vi "Open Command Panel.vi"(9 "Cached Commands":T1, 10 "Commands":cluster{"Time (s)":dbl, T2, bool}[](array[cluster]), 11 "Tag":string) -> (3 "Found":bool)   [LabVIEW 2025]
uses:
  Types/Single Cmd Info.ctl
  <vilib>/picture/picture.llb/imagedata.ctl
  Types/Command Editor Info.ctl
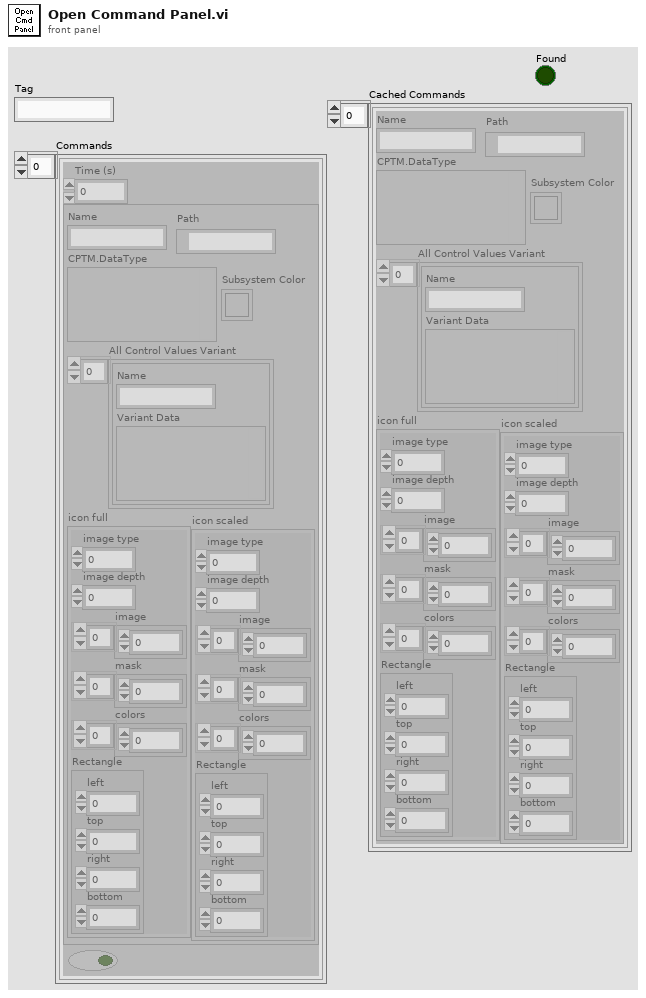
[diagram p1: front panel]
types:
  T1 = typedef "Command Editor Info.ctl" = T2[]
  T2 = typedef "Single Cmd Info.ctl" = cluster{"Name":string, "CPTM.DataType":variant, "All Control Values Variant":cluster{"Name":string, "Variant Data":variant}[], "icon full":T3, "icon scaled":T3, "Path":path, "Subsystem Color":u32}
  T3 = typedef "imagedata.ctl" = cluster{"image type":i32, "image depth":i32, "image":u8[], "mask":u8[], "colors":u32[], "Rectangle":cluster{"left":i16, "top":i16, "right":i16, "bottom":i16}}
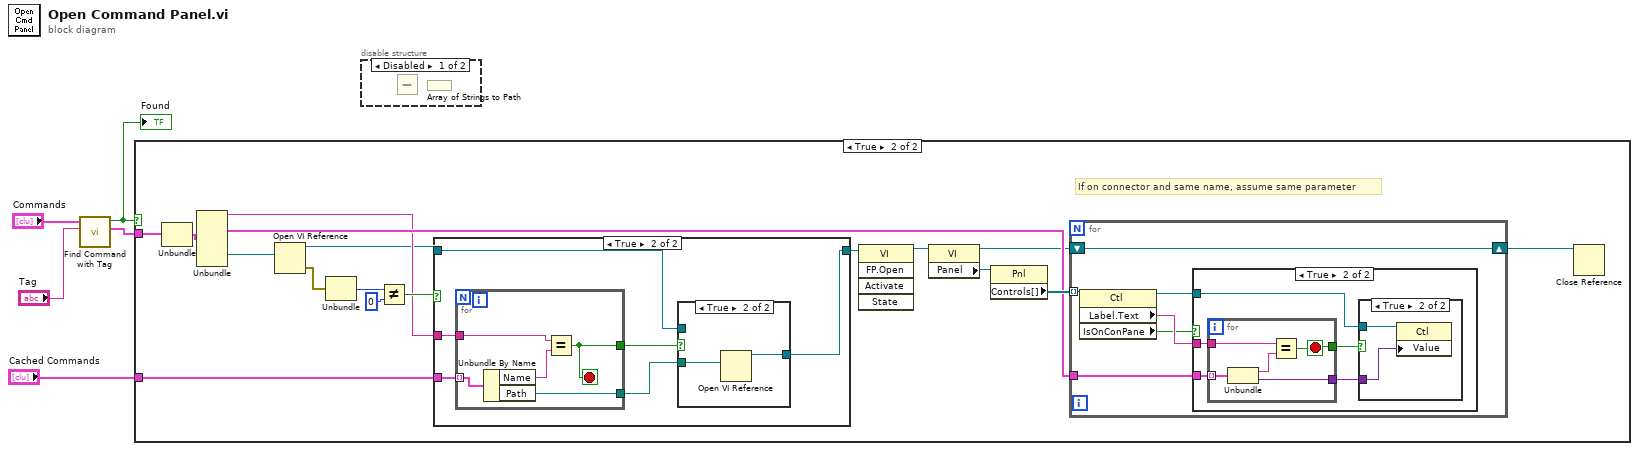
[diagram p0: block diagram]
diagram:
  n1 = call "Find Command with Tag.vi"("Command Tag"="Tag", "Commands"="Commands") -> ("Found Command"=w4:cluster{"Time (s)":dbl, T2, bool}, "Found"=w3:bool)  [unwired: 7 in, 1 out]
  "Found" <- w3
  n2 = case shown="True" w3 {
    tunnel: w4 -> [_ w22]
    tunnel: "Cached Commands" -> [_ w9]
    frame False {
    }
    frame True {
      # "If on connector and same name, assume same parameter"
      n3 = Unbundle(w22) -> (w21:T2)  [unwired: 2 out]
      n4 = Unbundle(w21) -> ("Name"=w8:string, "All Control Values Variant"=w17:cluster{"Name":string, "Variant Data":variant}[], "Path"=w11:path)  [unwired: 4 out]
      n5 = Open VI Reference(vi path=w11) -> (vi reference=w7:refnum<vi>, error out=w14:errorcluster)  [unwired: 5 in]
      n6 = Unbundle(w14) -> ("code"=w13:i32)  [unwired: 2 out]
      n7 = Not Equal?(x=w13, y=0) -> (x != y?=w10:bool)
      n8 = case shown="True" w10 {
        tunnel: w9 -> [_ w29]
        tunnel: w8 -> [_ w28]
        tunnel: w7 -> [w23 w24]
        tunnel: [w23 w25] -> w6
        frame False {
        }
        frame True {
          n9 = for {
            tunnel: w29 -> [w37] mode=indexing
            tunnel: w28 -> [w35]
            tunnel: [w34] -> w27
            tunnel: [w33] -> w26
            stop <- w34 stop-if-true
            n10 = Unbundle By Name(w37) -> ("Name"=w36:string, "Path"=w33:path)
            n11 = Equal?(x=w35, y=w36) -> (x = y?=w34:bool)
          }
          n12 = case shown="True" w27 {
            tunnel: w26 -> [_ w32]
            tunnel: [w30 w31] -> w25
            tunnel: w24 -> [w30 _]
            frame False {
            }
            frame True {
              n13 = Open VI Reference(vi path=w32) -> (vi reference=w31:refnum<vi>)  [unwired: 5 in, 1 out]
            }
          }
        }
      }
      n14 = invoke class="VI" method="FP.Open"(reference=w6) -> (reference out=w19:refnum<vi>)  [unwired: 4 in, 4 out]
      n15 = property class="VI"(reference=w19) -> (reference out=w16:refnum<vi>, "Panel"=w20:refnum<vi>)  [unwired: 1 in, 1 out]
      n16 = property class="Pnl"(reference=w20) -> ("Controls[]"=w18:refnum<vi>[])  [unwired: 1 in, 2 out]
      n17 = for {
        tunnel: w18 -> [w42] mode=indexing
        tunnel: w17 -> [w43]
        shift-right: [w38] -> w15
        shift-left: w16 -> [w38]
        n18 = property class="Ctl"(reference=w42) -> (reference out=w39:refnum<vi>, "Label.Text"=w41:string, "IsOnConPane"=w40:bool)  [unwired: 1 in, 1 out]
        n19 = case shown="True" w40 {
          tunnel: w43 -> [_ w48]
          tunnel: w41 -> [_ w47]
          tunnel: w39 -> [_ w46]
          frame False {
          }
          frame True {
            n20 = for {
              tunnel: w48 -> [w55] mode=indexing
              tunnel: [w54] -> w45
              tunnel: w47 -> [w53]
              tunnel: [w51] -> w44
              stop <- w51 stop-if-true
              n21 = Unbundle(w55) -> ("Name"=w52:string, "Variant Data"=w54:variant)
              n22 = Equal?(x=w53, y=w52) -> (x = y?=w51:bool)
            }
            n23 = case shown="True" w44 {
              tunnel: w46 -> [_ w50]
              tunnel: w45 -> [_ w49]
              frame False {
              }
              frame True {
                n24 = property class="Ctl"(reference=w50, "Value"=w49) -> ()  [unwired: 1 in, 2 out]
              }
            }
          }
        }
      }
      n25 = Close Reference(reference=w15) -> ()  [unwired: 1 in, 1 out]
    }
  }
  n26 = disable-structure shown="Disabled" {
    frame Disabled {
      n27 = Subtract() -> ()  [unwired: 2 in, 1 out]
      n28 = Array of Strings to Path() -> ()  [unwired: 2 in, 1 out]
    }
    frame Enabled {
    }
  }
